vi "Bearing between GPS pts.vi"(10 "Pt.2":T1={"Latitude"=2504.69148, "Longitude"=4361.44351} {"Longitude" format="%#_14g"; "Latitude" format="%#_14g"}, 11 "Pt.1":T1={"Latitude"=2504.69148, "Longitude"=4361.44351} {"Longitude" format="%#_14g"; "Latitude" format="%#_14g"}) -> (3 "Bearing Pt.1 to Pt.2":dbl)   [LabVIEW 2009]
uses:
  TypeDefs/Sensor Typedefs/GPS Data.ctl
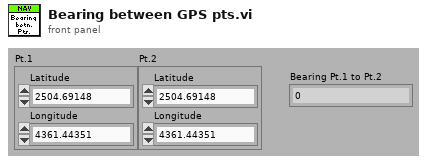
[diagram p1: front panel]
types:
  T1 = typedef "GPS Data.ctl" = cluster{"Latitude":dbl, "Longitude":dbl}
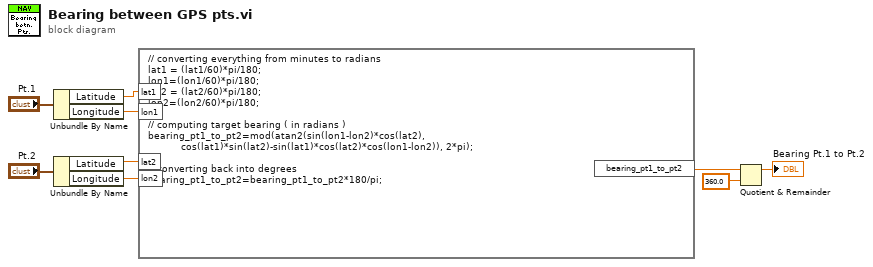
[diagram p0: block diagram]
diagram:
  n1 = Unbundle By Name("Pt.1") -> ("Latitude"=w9:dbl, "Longitude"=w8:dbl)
  n2 = Unbundle By Name("Pt.2") -> ("Latitude"=w7:dbl, "Longitude"=w6:dbl)
  n3 = formula code="// converting everything from minutes to radians\nlat1 = (lat1/60)*pi/180;\nlon1=(lon1/60)*pi/180;\nlat2 = (lat2/60)*pi/180;\nlon2=(lon2/60)*pi/180;\n\n// computing target bearing ( in radians )\nbearing_pt1_to_pt2=mod(atan2(sin(lon1-lon2)*cos(lat2),\n           cos(lat1)*sin(lat2)-sin(lat1)*cos(lat2)*cos(lon1-lon2)), 2*pi);\n\n// converting back into degrees\nbearing_pt1_to_pt2=bearing_pt1_to_pt2*180/pi;"("lon1"=w8, "lat1"=w9, "lat2"=w7, "lon2"=w6) -> ("bearing_pt1_to_pt2"=w5:dbl)
  n4 = Quotient & Remainder(x=w5, y=360.0) -> (x-y*floor(x/y)=→"Bearing Pt.1 to Pt.2":dbl)  [unwired: 1 out]
